vi "Create.vi"(10 "Group":refnum<class "Group.lvclass">) -> (3 "GroupValue out":refnum<class "GroupAbstractValue.lvclass">)   [LabVIEW 2020, in "Vecto.lvlib" / "GroupAbstractValue.lvclass"]
uses:
  GroupAbstractValue.lvclass
  Group/Group.lvclass
  GroupAbstractValue.lvclass/GroupAbstractValue.ctl
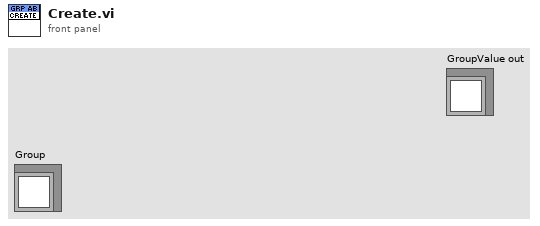
[diagram p1: front panel]
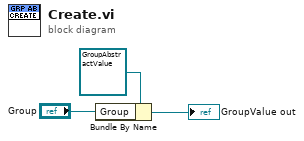
[diagram p0: block diagram]
diagram:
  n1 = Bundle By Name(cluster=refnum<class "GroupAbstractValue.lvclass"> refnum ("GroupValue out"), "Group"="Group") -> (→"GroupValue out":refnum<class "GroupAbstractValue.lvclass">)
